vi "DSF.Engine.Sequencer.Set Plugin Timings.vi"(8 "error in (no error)":errorcluster, 10 "Plugins":T1[](array[typedef]), 11 "Sequencer in":refnum<class "DSF.Engine.Sequencer.lvclass">) -> (0 "error out":errorcluster, 3 "Sequencer out":refnum<class "DSF.Engine.Sequencer.lvclass">)   [LabVIEW 2016, in "DSF.Engine.lvlib" / "DSF.Engine.Sequencer.lvclass"]
uses:
  DSF.Engine.Sequencer.lvclass
  DSF.Engine.Sequencer.Plugin.ctl
  Timing/DSF.Engine.Timing.lvclass
  DSF.Engine.Sequencer.lvclass/DSF.Engine.Sequencer.ctl
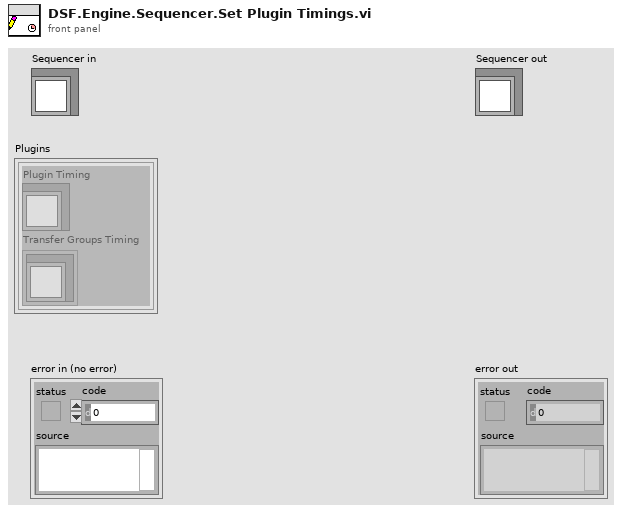
[diagram p1: front panel]
types:
  T1 = typedef "DSF.Engine.lvlib/DSF.Engine.Sequencer.lvclass/DSF.Engine.Sequencer.Plugin.ctl" = cluster{"Plugin Timing":refnum<class "DSF.Engine.Timing.lvclass">, "Transfer Groups Timing":refnum<class "DSF.Engine.Timing.lvclass">[]}
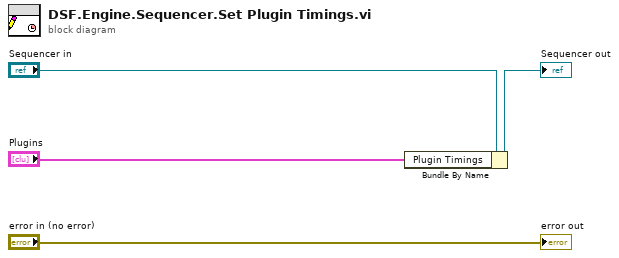
[diagram p0: block diagram]
diagram:
  n1 = Bundle By Name(cluster="Sequencer in", "Plugin Timings"="Plugins") -> (→"Sequencer out":refnum<class "DSF.Engine.Sequencer.lvclass">)
  "error out" <- "error in (no error)"
